vi "Write data.vi"(8 "error in (no error)":errorcluster, 10 "data":dbl[](array[numeric]), 11 "Plot_waveform in":refnum<class "Plot_waveform.lvclass">) -> (0 "error out":errorcluster, 3 "Plot_waveform out":refnum<class "Plot_waveform.lvclass">)   [LabVIEW 2019, in "Plot_waveform.lvclass"]
uses:
  Plot_waveform.lvclass
  Plot_waveform.lvclass/Plot_waveform.ctl
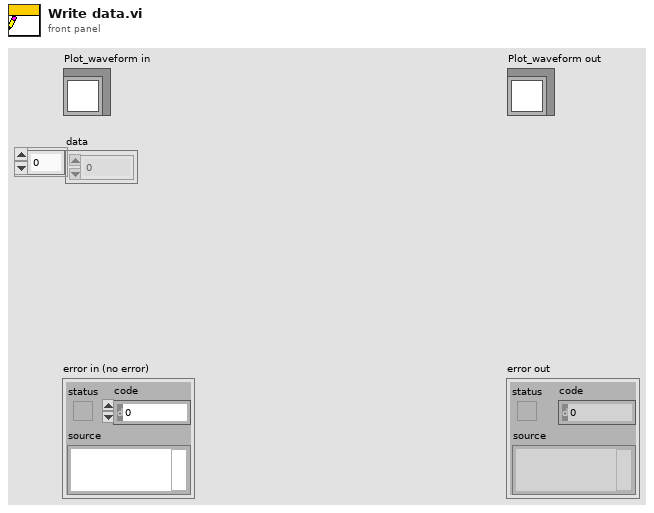
[diagram p1: front panel]
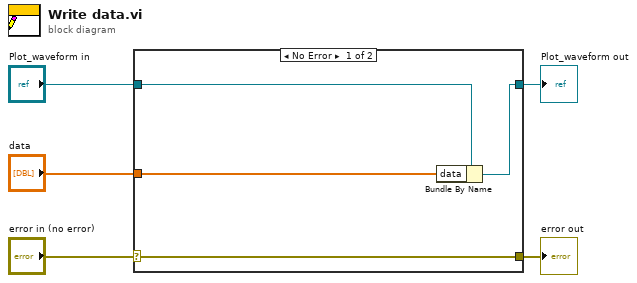
[diagram p0: block diagram]
diagram:
  n1 = case shown="No Error" "error in (no error)" {
    selector: "error in (no error)" -> [w9 w10]
    tunnel: [w9 w10] -> w4
    tunnel: [w7 w11] -> w2
    tunnel: "Plot_waveform in" -> [w8 w11]
    tunnel: "data" -> [w6 _]
    frame No Error {
      n2 = Bundle By Name(cluster=w8, "data"=w6) -> (w7:refnum<class "Plot_waveform.lvclass">)
    }
    frame Error {
    }
  }
  "error out" <- w4
  "Plot_waveform out" <- w2
